vi "Get Topologies (Device).vi"(8 "error in (no error)":errorcluster, 11 "device":refnum<k21>) -> (0 "error out":errorcluster, 3 "topologies":string[](array[string]))   [LabVIEW 2020, in "SLSC Switch.lvlib"]
doc: "Enumerates the possible SLSC Switch topologies."
uses:
  <vilib>/SLSC_Switch/SLSC Switch.lvlib
  nislscsl.dll
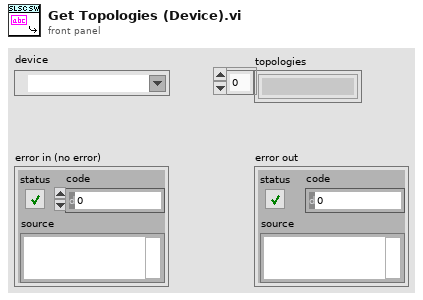
[diagram p1: front panel]
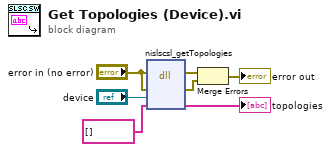
[diagram p0: block diagram]
diagram:
  n1 = dll-call lib="nislscsl.*" fn="nislscsl_getTopologies"(error in="error in (no error)", "errorCluster"="error in (no error)", "deviceIdentifier"="device", "topologies"=string[] [] ("array of strings")) -> (error out=w7:errorcluster, "errorCluster"=w6:errorcluster, "topologies"=→"topologies":string[])  [unwired: 4 in, 1 out]
  n2 = Merge Errors(w7, w6) -> (→"error out":errorcluster)
